vi "FPGA_small.vi"() -> ()   [LabVIEW 2018]
uses:
  <vilib>/Platform/TimedLoop/XDataNode/timing_clust.ctl
  <vilib>/Platform/TimedLoop/XDataNode/nitl_modes.ctl
  <vilib>/Platform/TimedLoop/XDataNode/wakeup.ctl
  <vilib>/rvi/Emulation/niFpgaGetClockAttributes.vi
  <vilib>/rvi/Emulation/niFpgaSctlEmulationGetInTimedLoop.vi
  <vilib>/rvi/Emulation/niFpgaEmulationReportErrorSimple.vi
  <vilib>/rvi/Emulation/niFpgaProcessEmulError.vi
  <vilib>/rvi/eio/common/nirviEmuTemplateMethod_errors.vi
  <vilib>/rvi/Emulation/niFpgaCriticalErrorInLSC.vi
  <vilib>/eio/EIONode/EIONode.xnode
  <vilib>/platform/TimedLoop/XDataNode/XDataNode.xnode
  <vilib>/Platform/TimedLoop/XDataNode/XDNodeRunTimeDep.lvlib
panel:
  in  "dir":bool
  in  "stop":bool
  out "speed":i16
  out "AI0":u16=1344
  out "dAI":i16=8
  in  "delayai_ms":u32=10
  in  "pwm_val":u32=1000
  in  "dt_pwm_ms":u32=300 caption="Count(uSec)"
  out "busy":bool
  in  "dt_cmd_us":u32=1 caption="delay_M_ms"
  out "backward":bool
  out "pos":i16=1241
  out "err cnt":i16
  in  "reset":bool
  out "off_track":bool
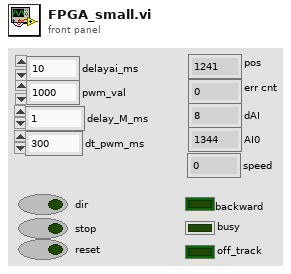
[diagram p1: front panel]
types:
  T1 = typedef "XDNodeRunTimeDep.lvlib/timing_clust.ctl" = cluster{"Expected End [f-1]":u64, "Actual End [f-1]":u64, "Finished Late? [f-1]":bool, "Expected End [i-1]":u64, "Actual End [i-1]":u64, "Finished Late? [i-1]":bool, "Expected Start [i]":u64, "Actual Start [i]":u64, "Expected Start [f]":u64, "Actual Start [f]":u64, "Source Name":string, "Structure Name":string, "Period":i64, "Deadline":i64, "Offset":i64, "Start":i64, "Priority":i32, "Timeout":i32, "Mode":T2, "Wakeup Reason":T3, "Error":errorcluster, "Source Type":string, "Secondary Source Type":string, "Global End Time":u64, "Global Start Time":u64, "Frame Duration":u64, "Iteration Duration":u64, "Assigned CPU":i32, "I/O Scan Engine Mode":u32}
  T2 = typedef "XDNodeRunTimeDep.lvlib/nitl_modes.ctl" = enum32{"No Change", "Process missed periods, maintain original phase", "Discard missed periods, maintain original phase", "Process missed periods, ignore original phase", "Discard missed periods, ignore original phase"}
  T3 = typedef "XDNodeRunTimeDep.lvlib/wakeup.ctl" = enum32{"Normal", "Aborted", "Asynchronous wakeup", "Timing source error", "Timed loop error", "Timeout"}
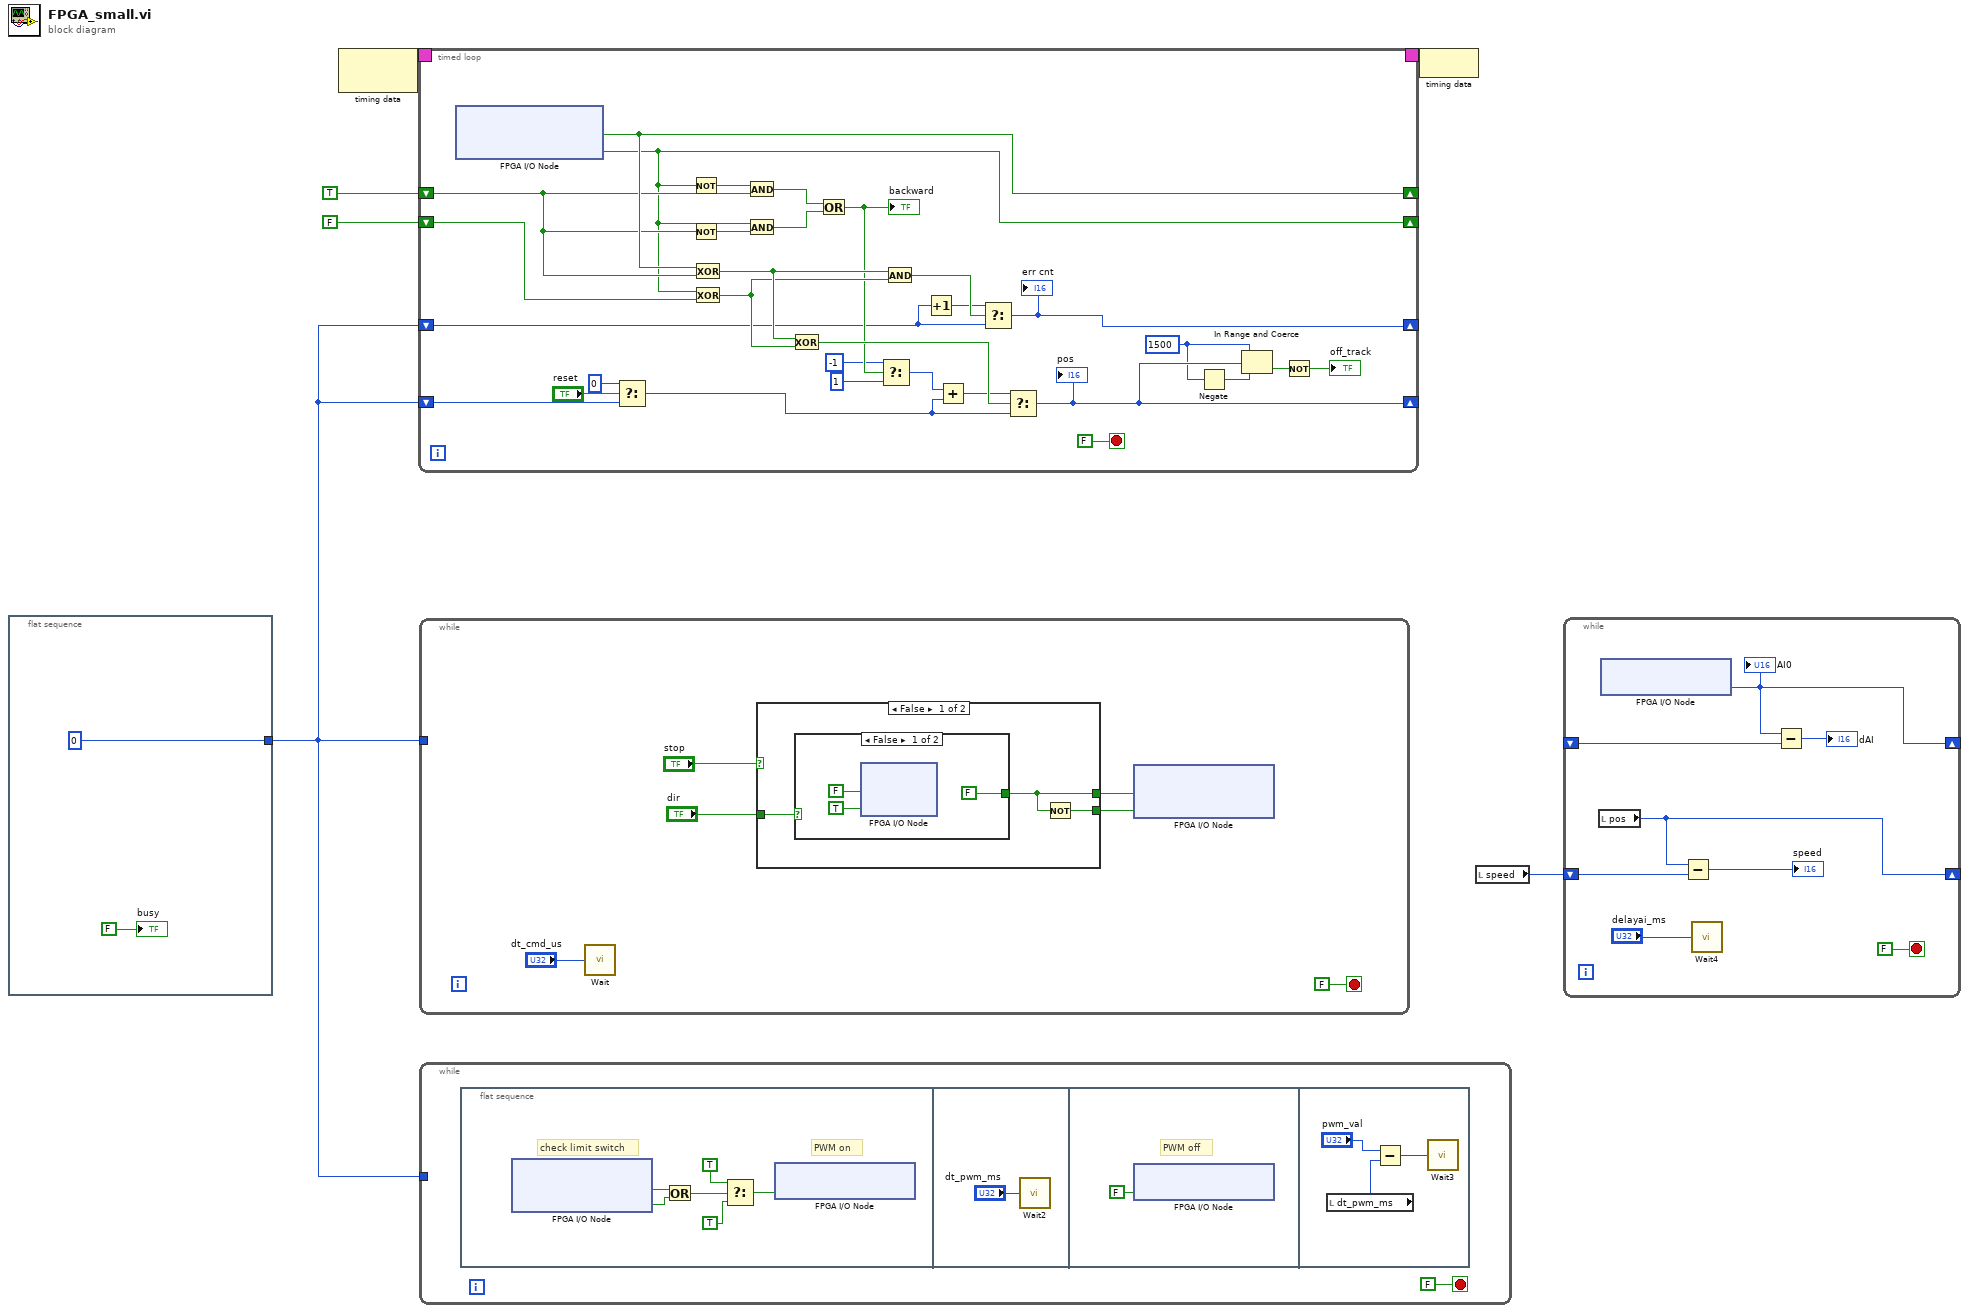
[diagram p0: block diagram]
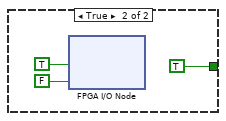
[diagram p2: hidden frame]
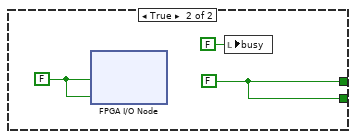
[diagram p3: hidden frame]
diagram:
  n1 = flat-sequence {
    tunnel: [i16 0] -> w1
    frame #0 {
      "busy" <- FALSE ("status")
    }
  }
  n2 = node-c288() -> (w6:T1)  [unwired: 1 in]
  n3 = timed-loop {
    timing: w6 -> [_]
    timing-out: [_] -> w5
    shift-right: [w33] -> _
    shift-left: TRUE ("ConnectorA/DIO11") -> [w32]
    shift-right: [w31] -> _
    shift-left: FALSE ("ConnectorA/DIO12") -> [w30]
    shift-right: [w13] -> _
    shift-left: w1 -> [w16]
    shift-right: [w18] -> _
    shift-left: w1 -> [w19]
    stop <- FALSE stop-if-true
    w9 = i16 1500 ("upper limit")
    n4 = xnode "FPGA I/O Node"() -> ("ConnectorA/DIO11"=w33:bool, "ConnectorA/DIO12"=w31:bool)  [unwired: 2 in, 2 out]
    n5 = Select(t=i16 0, s="reset", f=w16) -> (s? t:f=w14:i16)
    n6 = Not(x=w31) -> (.not. x?=w37:bool)
    n7 = Not(x=w32) -> (.not. x?=w36:bool)
    n8 = Exclusive Or(1:w32, 2:w33) -> (0:w29:bool)
    n9 = Exclusive Or(1:w30, 2:w31) -> (0:w28:bool)
    n10 = And(x=w37, y=w32) -> (x .and. y?=w34:bool)
    n11 = And(x=w31, y=w36) -> (x .and. y?=w35:bool)
    n12 = Exclusive Or(1:w28, 2:w29) -> (0:w27:bool)
    n13 = Or(x=w34, y=w35) -> (x .or. y?=w26:bool)
    "backward" <- w26
    n14 = Select(t=i16 -1, s=w26, f=i16 1) -> (s? t:f=w23:i16)
    n15 = And(x=w29, y=w28) -> (x .and. y?=w21:bool)
    n16 = Increment(x=w19) -> (x+1=w20:i16)
    n17 = Add(x=w23, y=w14) -> (x+y=w22:i16)
    n18 = Select(t=w20, s=w21, f=w19) -> (s? t:f=w18:i16)
    "err cnt" <- w18
    n19 = Select(t=w22, s=w27, f=w14) -> (s? t:f=w13:i16)
    "pos" <- w13
    n20 = Negate(x=w9) -> (-x=w10:i16)
    n21 = In Range and Coerce(upper limit=w9, x=w13, lower limit=w10) -> (In Range?=w12:bool)  [unwired: 1 out]
    n22 = Not(x=w12) -> (.not. x?=→"off_track":bool)
  }
  n23 = while {
    tunnel: w1 -> [_]
    stop <- FALSE stop-if-true
    n24 = call "Wait"("Count(uSec)"="dt_cmd_us") -> ()  [unwired: 1 out]
    n25 = case shown="False" "stop" {
      tunnel: [w49 w58] -> w44
      tunnel: [w48 w58] -> w43
      tunnel: "dir" -> [w47 _]
      frame False {
        n26 = case shown="False" w47 {
          tunnel: [FALSE ("dir") TRUE ("dir")] -> w48
          frame False {
            n27 = xnode "FPGA I/O Node"("LED0"=FALSE, "LED1"=TRUE) -> ()  [unwired: 2 in, 2 out]
          }
          frame True {
            n28 = xnode "FPGA I/O Node"("LED0"=TRUE, "LED1"=FALSE) -> ()  [unwired: 2 in, 2 out]
          }
        }
        n29 = Not(x=w48) -> (.not. x?=w49:bool)
      }
      frame True {
        w56 = FALSE ("LED0")
        w58 = FALSE ("dir")
        n30 = xnode "FPGA I/O Node"("LED0"=w56, "LED1"=w56) -> ()  [unwired: 2 in, 2 out]
        n31 = local write "busy"(FALSE ("busy")) -> ()
      }
    }
    n32 = xnode "FPGA I/O Node"("ConnectorA/DIO6"=w43, "ConnectorA/DIO5"=w44) -> ()  [unwired: 2 in, 2 out]
  }
  n33 = while {
    tunnel: w1 -> [_]
    stop <- FALSE stop-if-true
    n34 = flat-sequence {
      frame #0 {
        # "check limit switch"
        # "PWM on"
        n35 = xnode "FPGA I/O Node"() -> ("ConnectorA/DIO0"=w64:bool, "ConnectorA/DIO1"=w65:bool)  [unwired: 2 in, 2 out]
        n36 = Or(x=w64, y=w65) -> (x .or. y?=w63:bool)
        n37 = Select(t=TRUE, s=w63, f=TRUE ("ConnectorA/DIO8")) -> (s? t:f=w62:bool)
        n38 = xnode "FPGA I/O Node"("ConnectorA/DIO8"=w62) -> ()  [unwired: 1 in, 1 out]
      }
      frame #1 {
        n39 = call "Wait2"("Count(uSec)"="dt_pwm_ms") -> ()  [unwired: 1 out]
      }
      frame #2 {
        # "PWM off"
        n40 = xnode "FPGA I/O Node"("ConnectorA/DIO8"=FALSE) -> ()  [unwired: 1 in, 1 out]
      }
      frame #3 {
        n41 = local read "dt_pwm_ms"() -> (w70:u32)
        n42 = Subtract(x="pwm_val", y=w70) -> (x-y=w68:u32)
        n43 = call "Wait3"("Count(uSec)"=w68) -> ()  [unwired: 1 out]
      }
    }
  }
  n44 = node-c288(w5) -> ()
  n45 = local read "speed"() -> (w2:i16)
  n46 = while {
    shift-right: [w76] -> _
    shift-left: w2 -> [w75]
    shift-right: [w72] -> _
    shift-left: _ -> [w73]
    stop <- FALSE stop-if-true
    n47 = local read "pos"() -> (w76:i16)
    n48 = xnode "FPGA I/O Node"() -> ("ConnectorA/AI0"=w72:u16)  [unwired: 1 in, 1 out]
    "AI0" <- w72
    n49 = Subtract(x=w76, y=w75) -> (x-y=→"speed":i16)
    n50 = call "Wait4"("Count(mSec)"="delayai_ms") -> ()  [unwired: 1 out]
    n51 = Subtract(x=w72, y=w73) -> (x-y=→"dAI":u16)
  }
